vi "Validate.vi"(8 "error in":errorcluster, 10 "parameters":variant, 11 "NISE_CEF_HierarchyRepo in":refnum<class "NISE_CEF_HierarchyRepo.lvclass">) -> (0 "error out":errorcluster, 3 "NISE_CEF_HierarchyRepo out":refnum<class "NISE_CEF_HierarchyRepo.lvclass">)   [LabVIEW 2013, in "NISE_CEF_HierarchyRepo.lvclass"]
uses:
  NISE_CEF_HierarchyRepo.lvclass
  NISE_CEF_HierarchyRepo.lvclass/NISE_CEF_HierarchyRepo.ctl
  serializable configuration/NISE_CEF_serializable configuration.lvclass
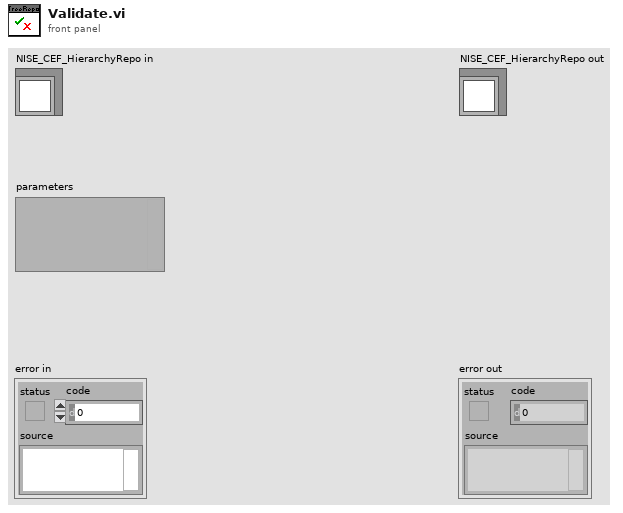
[diagram p1: front panel]
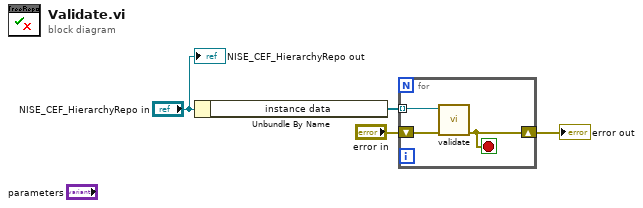
[diagram p0: block diagram]
diagram:
  n1 = Unbundle By Name("NISE_CEF_HierarchyRepo in") -> ("instance data"=w1:refnum<class "NISE_CEF_serializable configuration.lvclass">[])
  n2 = for {
    shift-right: [w6] -> w2
    shift-left: "error in" -> [w7]
    tunnel: w1 -> [w5] mode=indexing
    stop <- w6 stop-if-true
    n3 = call-dynamic "validate.vi"("error in"=w7, "configuration in"=w5) -> ("error out"=w6:errorcluster)  [unwired: 8 in, 1 out]
  }
  "error out" <- w2
  "NISE_CEF_HierarchyRepo out" <- "NISE_CEF_HierarchyRepo in"
